vi "ReserveCDAQDevice.vi"(8 "error in (no error)":errorcluster, 11 "cDAQ Device":tag) -> (0 "error out":errorcluster, 2 "Force close":string, 3 "device out":tag)   [LabVIEW 2018, in "Acquisition.lvlib"]
uses:
  Acquisition.lvlib
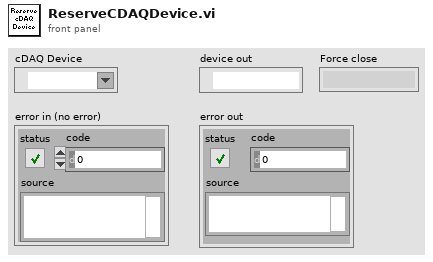
[diagram p1: front panel]
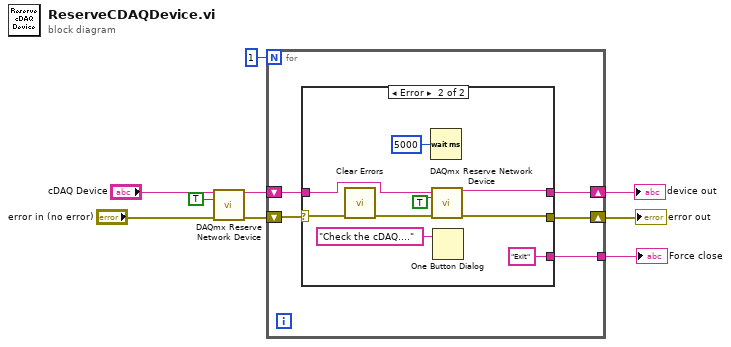
[diagram p0: block diagram]
diagram:
  n1 = call <vilib>:"DAQmx Reserve Network Device.vi"("device in"="cDAQ Device", "override reservation?"=TRUE, "error in"="error in (no error)") -> ("device out"=w3:tag, "error out"=w2:errorcluster)  [unwired: 11 in]
  n2 = for {
    N: 1 -> [_]
    shift-right: [w14] -> w6
    shift-left: w3 -> [w12]
    shift-right: [w13] -> w5
    shift-left: w2 -> [w11]
    tunnel: [w10] -> w1
    n3 = case shown="Error" w11 {
      selector: w11 -> [w15 w23]
      tunnel: w12 -> [w16 w19]
      tunnel: [w16 w20] -> w14
      tunnel: [w15 w21] -> w13
      tunnel: [_ "Exit"] -> w10
      frame No Error {
      }
      frame Error {
        n4 = call <vilib>:"Clear Errors.vi"("error in (no error)"=w23) -> ("error out"=w22:errorcluster)  [unwired: 5 in, 1 out]
        n5 = Wait (ms)(milliseconds to wait=u32 5000) -> ()  [unwired: 1 out]
        n6 = call <vilib>:"DAQmx Reserve Network Device.vi"("device in"=w19, "override reservation?"=TRUE, "error in"=w22) -> ("device out"=w20:tag, "error out"=w21:errorcluster)  [unwired: 11 in]
        n7 = One Button Dialog(message="Check the cDAQ....") -> ()  [unwired: 1 in, 1 out]
      }
    }
  }
  "device out" <- w6
  "error out" <- w5
  "Force close" <- w1
